vi "Read EndGame_.vi"(8 "error in (no error)":errorcluster, 11 "SnakeSwitch in":refnum<class "SnakeSwitch.lvclass">) -> (0 "error out":errorcluster, 2 "EndGame?":bool, 3 "SnakeSwitch out":refnum<class "SnakeSwitch.lvclass">)   [LabVIEW 2019, in "RT_Game.lvlib" / "SnakeSwitch.lvclass"]
uses:
  SnakeSwitch.lvclass
  SnakeSwitch.lvclass/SnakeSwitch.ctl
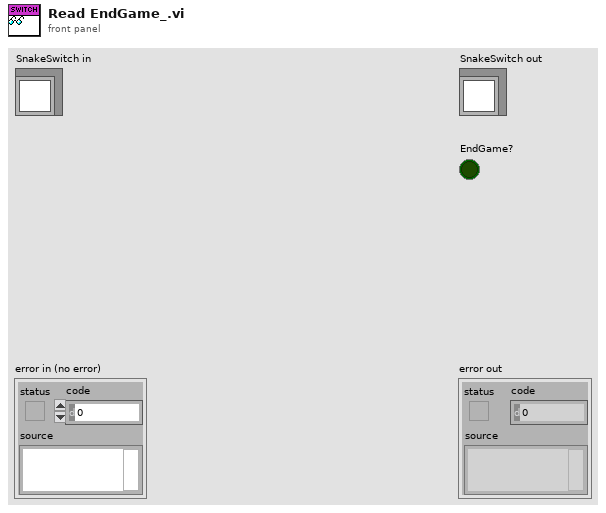
[diagram p1: front panel]
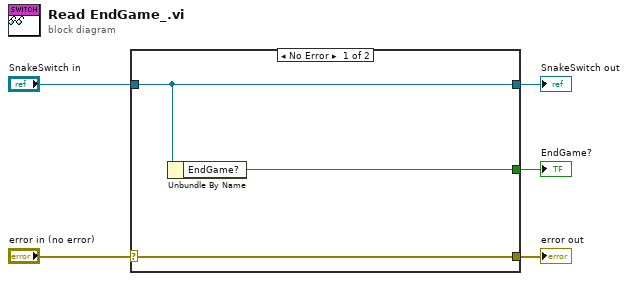
[diagram p0: block diagram]
diagram:
  n1 = case shown="No Error" "error in (no error)" {
    selector: "error in (no error)" -> [w8 w9]
    tunnel: [w8 w9] -> w4
    tunnel: [w7 w10] -> w2
    tunnel: "SnakeSwitch in" -> [w7 w10]
    tunnel: [w6 _] -> w1
    frame No Error {
      n2 = Unbundle By Name(w7) -> ("EndGame?"=w6:bool)
    }
    frame Error {
    }
  }
  "error out" <- w4
  "SnakeSwitch out" <- w2
  "EndGame?" <- w1
